vi "Get Current Font.vi"(0 "report in":refnum<class "NI_report.lvclass">, 11 "error in (no error)":errorcluster) -> (4 "report.lvclass":refnum<class "NI_report.lvclass">, 6 "font":T1, 15 "error out":errorcluster)   [LabVIEW 2017, in "NI_ReportGenerationToolkit.lvlib"]
uses:
  <vilib>/addons/_office/NI_ReportGenerationToolkit.lvlib
  <vilib>/Utility/NIReport.llb/NI_report.lvclass
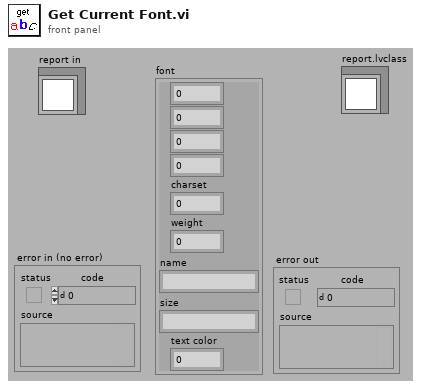
[diagram p1: front panel]
types:
  T1 = cluster{i32, i32, i32, i32, "charset":i16, "weight":i16, "name":string, "size":string, "text color":u32}
  T2 = cluster{"Italic":bool, "StrikeThrough":bool, "Underline":bool, "Bold":bool}
  T3 = cluster{"charset":i16, "name":string, "weight":i16, "size":string}
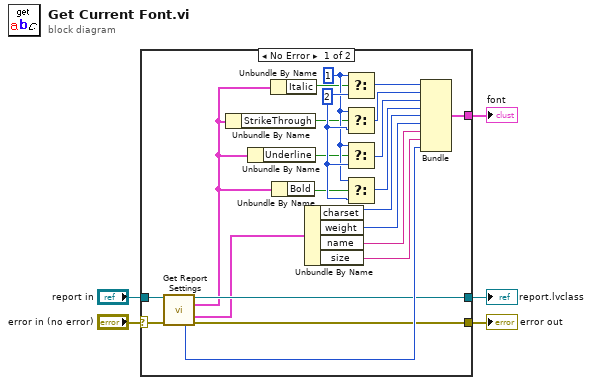
[diagram p0: block diagram]
diagram:
  n1 = case shown="No Error" "error in (no error)" {
    selector: "error in (no error)" -> [w6 w28]
    tunnel: [w27 _] -> w5
    tunnel: [w17 w29] -> w4
    tunnel: "report in" -> [w16 w29]
    tunnel: [w14 w28] -> w2
    frame No Error {
      w12 = 1
      w13 = 2
      n2 = call-dynamic "Get Report Settings.vi"("report in"=w16, "error in (no error)"=w6) -> ("report out"=w17:refnum<class "NI_report.lvclass">, "text options"=w7:T2, "font settings"=w15:T3, "text color"=w26:u32, "error out"=w14:errorcluster)  [unwired: 9 in]
      n3 = Unbundle By Name(w7) -> ("StrikeThrough"=w9:bool)
      n4 = Unbundle By Name(w7) -> ("Underline"=w10:bool)
      n5 = Unbundle By Name(w7) -> ("Italic"=w8:bool)
      n6 = Unbundle By Name(w7) -> ("Bold"=w11:bool)
      n7 = Unbundle By Name(w15) -> ("charset"=w22:i16, "weight"=w23:i16, "name"=w24:string, "size"=w25:string)
      n8 = Select(t=w12, s=w8, f=w13) -> (s? t:f=w18:i32)
      n9 = Select(t=w12, s=w9, f=w13) -> (s? t:f=w19:i32)
      n10 = Select(t=w12, s=w10, f=w13) -> (s? t:f=w20:i32)
      n11 = Select(t=w12, s=w11, f=w13) -> (s? t:f=w21:i32)
      n12 = Bundle(w18, w19, w20, w21, "charset"=w22, "weight"=w23, "name"=w24, "size"=w25, "text color"=w26) -> (w27:T1)  [unwired: 1 in]
    }
    frame Error {
    }
  }
  "font" <- w5
  "report.lvclass" <- w4
  "error out" <- w2
